vi "CalculateFrames_v02.vi"(8 "Program Spin Coater":T1(array[cluster]), 9 "Seconds End":dbl[unit], 10 "Seconds Start":dbl[unit], 11 "Frame Rate":dbl[unit]) -> (1 "Time":dbl, 2 "Frames":i32)   [LabVIEW 2020]
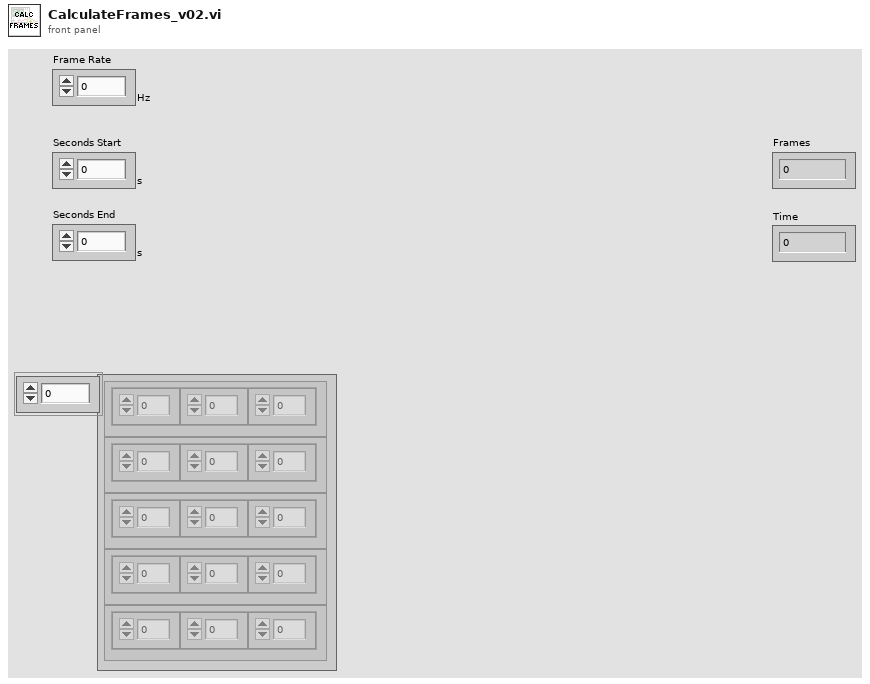
[diagram p1: front panel]
types:
  T1 = cluster{"Speed (rpm)":dbl, "Time (s)":dbl, "Acc (rpm/s)":dbl}[]
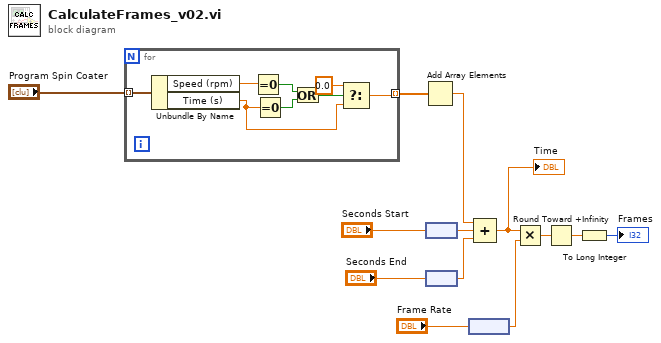
[diagram p0: block diagram]
diagram:
  n1 = for {
    tunnel: "Program Spin Coater" -> [w21] mode=indexing
    tunnel: [w14] -> w1 mode=indexing
    n2 = Unbundle By Name(w21) -> ("Speed (rpm)"=w20:dbl, "Time (s)"=w16:dbl)
    n3 = Equal To 0?(x=w20) -> (x = 0?=w19:bool)
    n4 = Equal To 0?(x=w16) -> (x = 0?=w18:bool)
    n5 = Or(x=w19, y=w18) -> (x .or. y?=w17:bool)
    n6 = Select(t=0.0, s=w17, f=w16) -> (s? t:f=w14:dbl)
  }
  n7 = Add Array Elements(numeric array=w1) -> (sum=w13:dbl)
  n8 = node("Seconds Start") -> (w11:dbl)
  n9 = node("Seconds End") -> (w9:dbl)
  n10 = node("Frame Rate") -> (w6:dbl)
  n11 = Compound Arithmetic op=ADD(w13, w11, w9) -> (w8:dbl)
  "Time" <- w8
  n12 = Multiply(x=w8, y=w6) -> (x*y=w5:dbl)
  n13 = Round Toward +Infinity(x=w5) -> (ceil(x): smallest int >= x=w4:dbl)
  n14 = To Long Integer(number=w4) -> (32bit integer=→"Frames":i32)
